vi "case structure for led boxes.vi"() -> ()   [LabVIEW 2016]
panel:
  out "RED":bool
  out "YELLOW":bool
  out "GREEN":bool
  out "BLUE":bool
  in  "Color Selector":enum16{"RED", "GREEN", "BLUE", "YELLOW"}(ring)
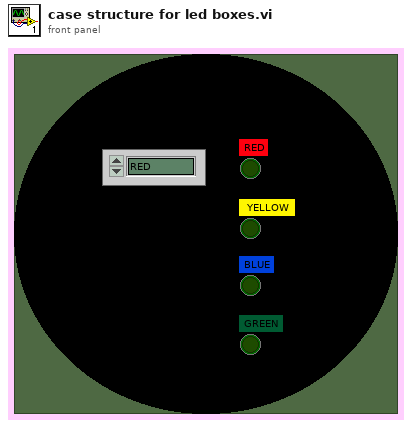
[diagram p1: front panel]
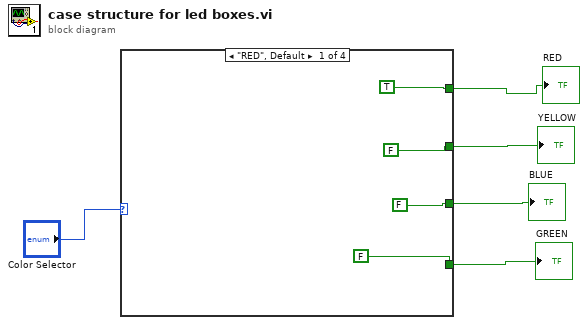
[diagram p0: block diagram]
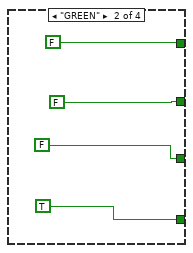
[diagram p2: hidden frame]
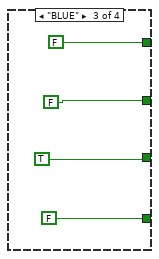
[diagram p3: hidden frame]
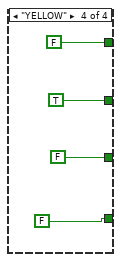
[diagram p4: hidden frame]
diagram:
  n1 = case shown="\"RED\", Default" "Color Selector" {
    tunnel: [FALSE TRUE FALSE FALSE] -> w4
    tunnel: [FALSE FALSE FALSE TRUE] -> w3
    tunnel: [TRUE FALSE FALSE FALSE] -> w2
    tunnel: [FALSE FALSE TRUE FALSE] -> w1
    frame "RED", Default {
    }
    frame "GREEN" {
    }
    frame "BLUE" {
    }
    frame "YELLOW" {
    }
  }
  "BLUE" <- w1
  "GREEN" <- w4
  "YELLOW" <- w3
  "RED" <- w2
